vi "GA Get Trap Prm Single.vi"(0 "nAxisNum":i16, 1 "dSmoothTime":i16, 5 "dAcc":dbl, 7 "dDec":dbl, 9 "dVelStart":dbl, 11 "error in (no error)":errorcluster caption="错误输入（无错误）") -> (3 "dSmoothTime out":i16, 4 "function return":i32, 6 "dAcc out":dbl, 8 "dDec out":dbl, 10 "dVelStart out":dbl, 15 "error out":errorcluster caption="错误输出")   [LabVIEW 2015, in "GAS.lvlib"]
doc: "extern \"C\" __declspec(dllimport) int GA_GetTrapPrmSingle(short nAxisNum,double* dAcc,double* dDec,double* dVelStart,short* dSmoothTime);"
uses:
  <userlib>/BP_GAS/GAS.lvlib
  <userlib>/BP_GAS/GAS.dll
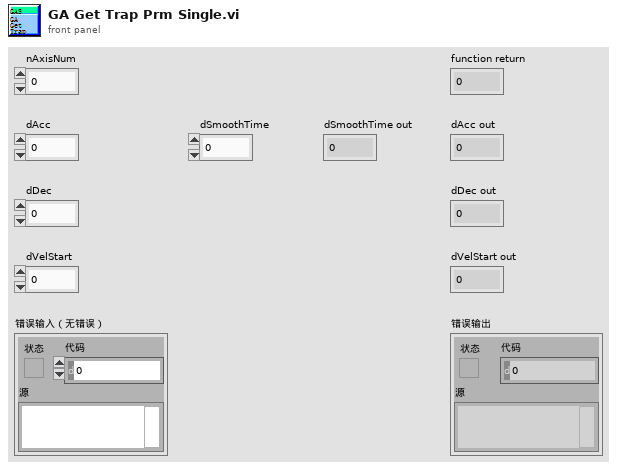
[diagram p1: front panel]
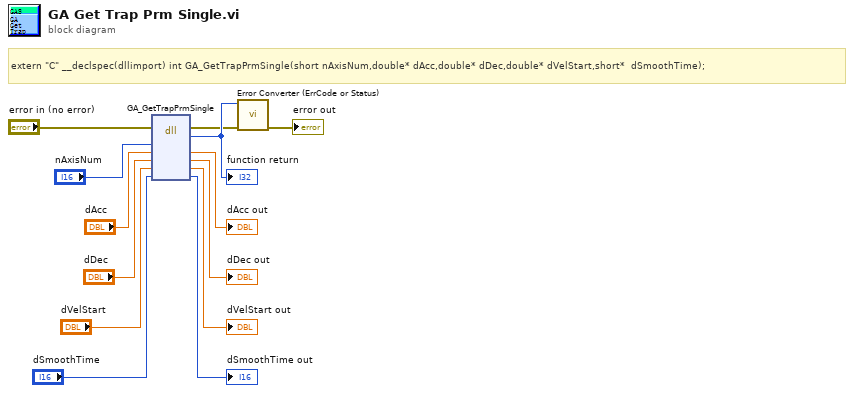
[diagram p0: block diagram]
diagram:
  # "extern \"C\" __declspec(dllimport) int GA_GetTrapPrmSingle(short nAxisNum,double* dAcc,double* dDec,double* dVelStart,short*  dSmoothTime);"
  n1 = dll-call lib="E:/Program Files (x86)/National Instruments/LabVIEW 2015/user.lib/BP_GAS/GAS.*" fn="GA_GetTrapPrmSingle"(error in="error in (no error)", "nAxisNum"="nAxisNum", "dAcc"="dAcc", "dDec"="dDec", "dVelStart"="dVelStart", "dSmoothTime"="dSmoothTime") -> (error out=w2:errorcluster, w13:i32, "dAcc"=→"dAcc out":dbl, "dDec"=→"dDec out":dbl, "dVelStart"=→"dVelStart out":dbl, "dSmoothTime"=→"dSmoothTime out":i16)  [unwired: 3 in, 1 out]
  "function return" <- w13
  n2 = call "Error Converter (ErrCode or Status).vi"("error in (no error)"=w2, "error code"=w13) -> ("error out"=→"error out":errorcluster)  [unwired: 9 in]
